vi "equal.vi"() -> ()   [LabVIEW 2019]
panel:
  out "x = y?":bool
  in  "data 2":dbl
  in  "data 1":dbl
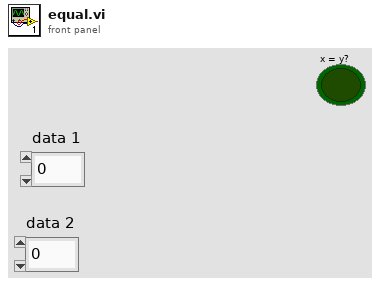
[diagram p1: front panel]
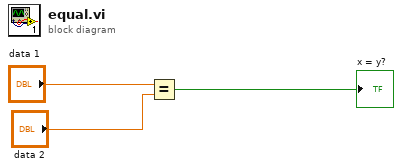
[diagram p0: block diagram]
diagram:
  n1 = Equal?(x="data 1", y="data 2") -> (x = y?=→"x = y?":bool)
